vi "test_character count _GT.vi"(8 "error in (no error)":errorcluster, 11 "TestCase in":refnum<class "Return Response Triggers.lvclass">) -> (0 "error out":errorcluster, 3 "TestCase out":refnum<class "Return Response Triggers.lvclass">)   [LabVIEW 2017, in "Return Response Triggers.lvclass"]
uses:
  Return Response Triggers.lvclass
  Libraries/SSH/Return Request Configuration.ctl
  Libraries/SSH/Response Configuration.ctl
  Libraries/SSH/Expected Response String Config.ctl
  Libraries/SSH/Search Start Point.ctl
  Libraries/SSH/Character Count Configuration.ctl
  <vilib>/addons/_JKI Toolkits/VI Tester/TestCase.llb/TestCase.lvclass
  Libraries/SSH/SSH.lvlib
  C:/Program Files (x86)/National Instruments/LabVIEW 2017/vi.lib/addons/_JKI Toolkits/VI Tester/TestCase.llb/TestCase.lvclass
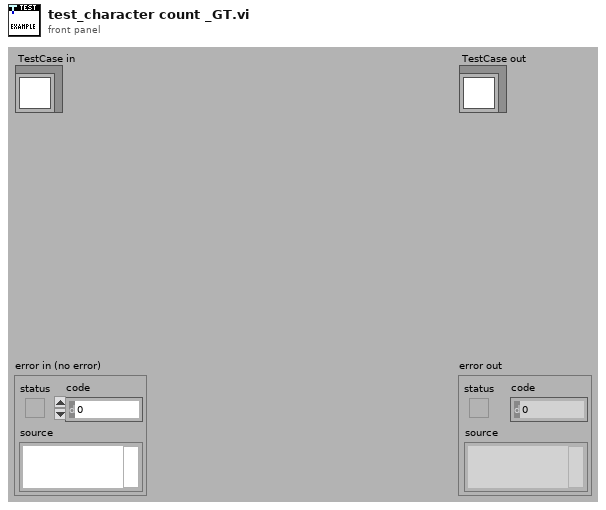
[diagram p1: front panel]
types:
  T1 = typedef "SSH.lvlib/Return Request Configuration.ctl" = cluster{"Response Configuration":T2, "Return Notifier":refnum<notifier>, "Response Requested":bool, "Command":string, "Initial Timer Value":u32, "Buffer Length":i32}
  T2 = typedef "SSH.lvlib/Response Configuration.ctl" = cluster{"Expected Response String":T3, "Character Count Config":T5, "Timeout (ms)":i32}
  T3 = typedef "SSH.lvlib/Expected Response String Config.ctl" = cluster{"Expected Response":string, "Search Start Point":T4, "Instance Count":i32}
  T4 = typedef "SSH.lvlib/Search Start Point.ctl" = enum16{"From Start", "From End"}
  T5 = typedef "SSH.lvlib/Character Count Configuration.ctl" = cluster{"Character Count Limit":i32, "Include Buffer":bool}
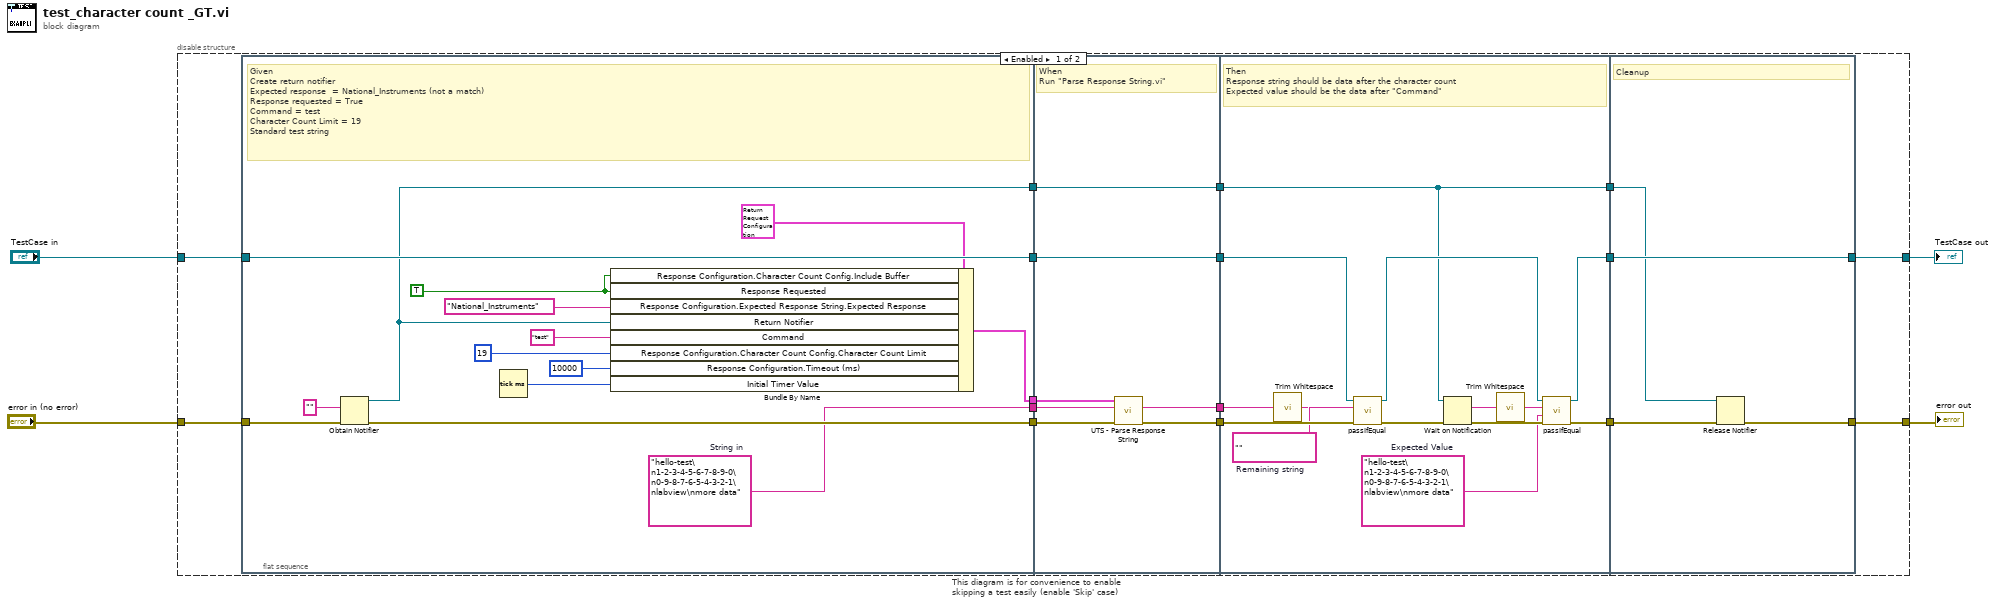
[diagram p0: block diagram]
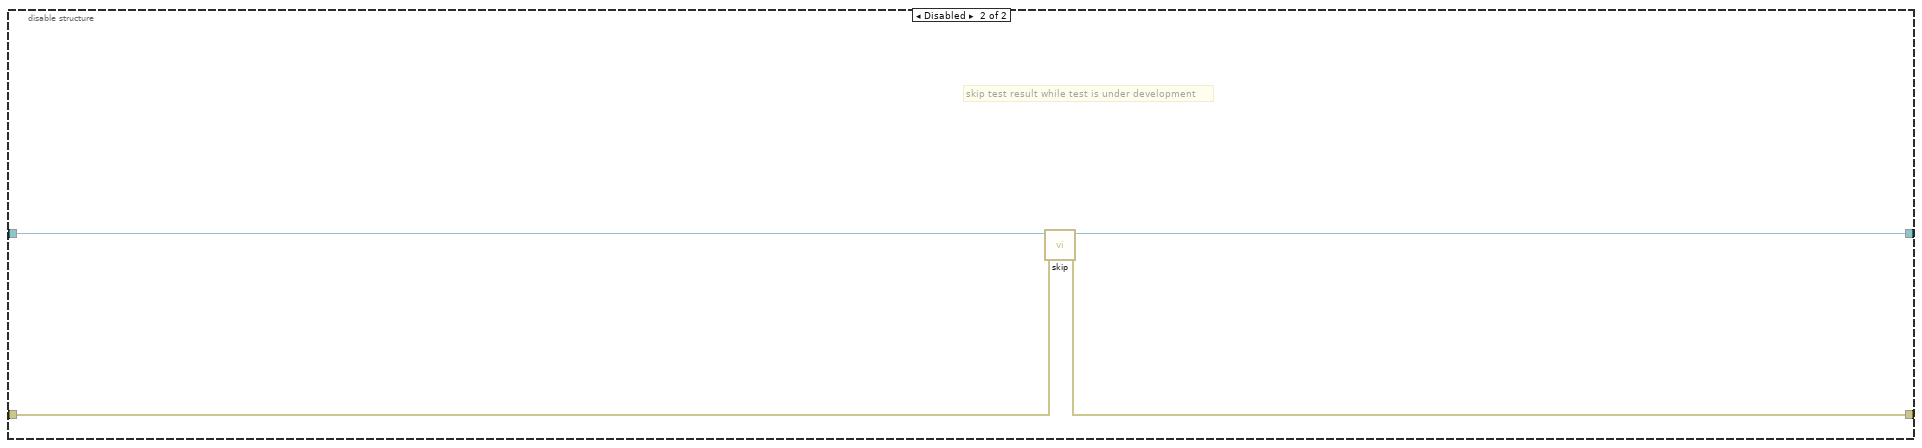
[diagram p2: hidden frame]
diagram:
  n1 = disable-structure "This diagram is for convenience to enable skipping a test easily (enable 'Skip' case)" shown="Enabled" {
    disable-tunnel: "TestCase in" -> [w13 w63]
    disable-tunnel: [w12 w61] -> w1
    disable-tunnel: [w11 w62] -> w3
    disable-tunnel: "error in (no error)" -> [w14 w60]
    frame Enabled {
      n2 = flat-sequence {
        tunnel: w14 -> [w31]
        tunnel: w13 -> [w34]
        tunnel: [w34] -> w20
        tunnel: [w30] -> w19
        tunnel: [w29] -> w10
        tunnel: [w26] -> w9
        tunnel: [w25] -> w8
        tunnel: [w41] -> w18
        tunnel: [w39] -> w17
        tunnel: w20 -> [w41]
        tunnel: w19 -> [w40]
        tunnel: w10 -> [w38]
        tunnel: w9 -> [w35]
        tunnel: w8 -> [w37]
        tunnel: [w36] -> w7
        tunnel: [w35] -> w6
        tunnel: [w48] -> w16
        tunnel: [w50] -> w15
        tunnel: w18 -> [w55]
        tunnel: w17 -> [w54]
        tunnel: w7 -> [w52]
        tunnel: w6 -> [w45]
        tunnel: [w45] -> w5
        tunnel: [w57] -> w11
        tunnel: [w59] -> w12
        tunnel: w16 -> [w59]
        tunnel: w15 -> [w58]
        tunnel: w5 -> [w56]
        frame #0 {
          w25 = "hello-test\n1-2-3-4-5-6-7-8-9-0\n0-9-8-7-6-5-4-3-2-1\nlabview\nmore data"  # String in
          w21 = TRUE ("Response Requested")
          # "Given\nCreate return notifier\nExpected response  = National_Instruments (not a match)\nResponse requested = True\nCommand = test\nCharacter Count Limit = 19\nStandard test string"
          n3 = Obtain Notifier(notification data type="", error in (no error)=w31) -> (notifier out=w26:refnum<notifier>, error out=w30:errorcluster)  [unwired: 2 in, 1 out]
          n4 = Tick Count (ms)() -> (millisecond timer value=w23:u32)
          n5 = Bundle By Name(cluster=T1 {"Response Configuration"={"Expected Response String"={"Expected Response"="", "Search Start Point"=enum."From Start", "Instance Count"=0}, "Character Count Config"={"Character Count Limit"=0, "Include Buffer"=FALSE}, "Timeout (ms)"=0}, "Return Notifier"=refnum, "Response Requested"=FALSE, "Command"="", "Initial Timer Value"=0, "Buffer Length"=0} ("Return Request in"), "Response Configuration.Character Count Config.Include Buffer"=w21, "Response Requested"=w21, "Response Configuration.Expected Response String.Expected Response"="National_Instruments" ("Response Configuration.Expected Response"), "Return Notifier"=w26, "Command"="test", "Response Configuration.Character Count Config.Character Count Limit"=19 ("Response Configuration.Character Count Limit"), "Response Configuration.Timeout (ms)"=10000, "Initial Timer Value"=w23) -> (w29:T1)
        }
        frame #1 {
          # "When\nRun \"Parse Response String.vi\""
          n6 = call "UTS - Parse Response String.vi"("error in (no error)"=w40, "Response String in"=w37, "Return Request in"=w38) -> ("error out"=w39:errorcluster, "Response String out"=w36:string)  [unwired: 6 in, 1 out]
        }
        frame #2 {
          w44 = ""  # Remaining string
          w47 = "hello-test\n1-2-3-4-5-6-7-8-9-0\n0-9-8-7-6-5-4-3-2-1\nlabview\nmore data"  # Expected Value
          # "Then\nResponse string should be data after the character count\nExpected value should be the data after \"Command\""
          n7 = call <vilib>:"Trim Whitespace.vi"("string"=w52) -> ("trimmed string"=w43:string)  [unwired: 1 in]
          n8 = call-dynamic "passIfEqual.vi"("error in (no error)"=w54, "y"=w44, "x"=w43, "TestCase in"=w55) -> ("error out"=w53:errorcluster, "TestCase out"=w49:refnum<class "Return Response Triggers.lvclass">)  [unwired: 6 in]
          n9 = Wait on Notification(notifier=w45, error in (no error)=w53) -> (notification=w46:string, error out=w51:errorcluster)  [unwired: 2 in, 2 out]
          n10 = call <vilib>:"Trim Whitespace.vi"("string"=w46) -> ("trimmed string"=w42:string)  [unwired: 1 in]
          n11 = call-dynamic "passIfEqual.vi"("error in (no error)"=w51, "y"=w47, "x"=w42, "TestCase in"=w49) -> ("error out"=w50:errorcluster, "TestCase out"=w48:refnum<class "Return Response Triggers.lvclass">)  [unwired: 6 in]
        }
        frame #3 {
          # "Cleanup"
          n12 = Release Notifier(notifier=w56, error in (no error)=w58) -> (error out=w57:errorcluster)  [unwired: 1 in, 2 out]
        }
      }
    }
    frame Disabled {
      # "skip test result while test is under development"
      n13 = call <vilib>:"skip.vi"("error in (no error)"=w60, "TestCase in"=w63) -> ("error out"=w62:errorcluster, "TestCase out"=w61:refnum<class "Return Response Triggers.lvclass">)  [unwired: 8 in]
    }
  }
  "error out" <- w3
  "TestCase out" <- w1
